vi "Describe Call Comparison.vi"(10 "VI Call 2":T1, 11 "VI Call 1":T1) -> (3 "delimited string":string)   [LabVIEW 2020, in "Matching String Input Comparator.lvclass"]
uses:
  Matching String Input Comparator.lvclass
  Core/Comparator/Comparator.lvclass
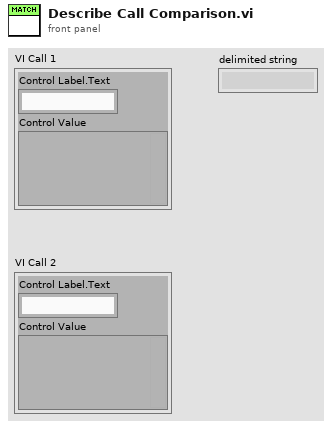
[diagram p1: front panel]
types:
  T1 = cluster{"Control Label.Text":string, "Control Value":variant}
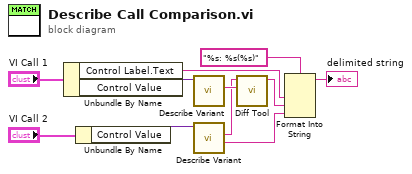
[diagram p0: block diagram]
diagram:
  n1 = Unbundle By Name("VI Call 1") -> ("Control Label.Text"=w7:string, "Control Value"=w10:variant)
  n2 = Unbundle By Name("VI Call 2") -> ("Control Value"=w9:variant)
  n3 = call "Describe Variant.vi"("Variant"=w10) -> ("Description"=w3:string)  [unwired: 8 in, 2 out]
  n4 = call "Describe Variant.vi"("Variant"=w9) -> ("Type Description"=w1:string, "Description"=w2:string)  [unwired: 8 in, 1 out]
  n5 = call "Diff Tool.vi"("Reference"=w3, "Target"=w2) -> ("Result"=w4:string)  [unwired: 8 in, 1 out]
  n6 = Format Into String(format string="%s: %s(%s)", w7, w4, w1) -> (resulting string=→"delimited string":string)  [unwired: 2 in, 1 out]
